vi "Drive Encoder Limit.vi"(0 "MotorControlDevRef":T1, 5 "MotorControlDevRef 2":T1, 7 "MotorControlDevRef 3":T1, 9 "MotorControlDevRef 4":T1, 11 "Limit":dbl, 12 "Invert":bool) -> (4 "MotorControlDevRef out":T1, 6 "MotorControlDevRef out 2":T1, 8 "MotorControlDevRef out 3":T1, 10 "MotorControlDevRef out 4":T1, 15 "Limit Triggered":bool)   [LabVIEW 2019]
uses:
  <vilib>/Rock Robotics/WPI/MotorControl/WPI_MotorControlDeviceRef.ctl
  <vilib>/Rock Robotics/WPI/MotorControl/WPI_MotorControlType.ctl
  <vilib>/Rock Robotics/SystemInterfaces/DIO/FPGA_DIOPWMChannel.ctl
  <vilib>/Rock Robotics/WPI/PWM/WPI_PWMDeadband.ctl
  <vilib>/Rock Robotics/SystemInterfaces/DIO/FPGA_DIOChannel.ctl
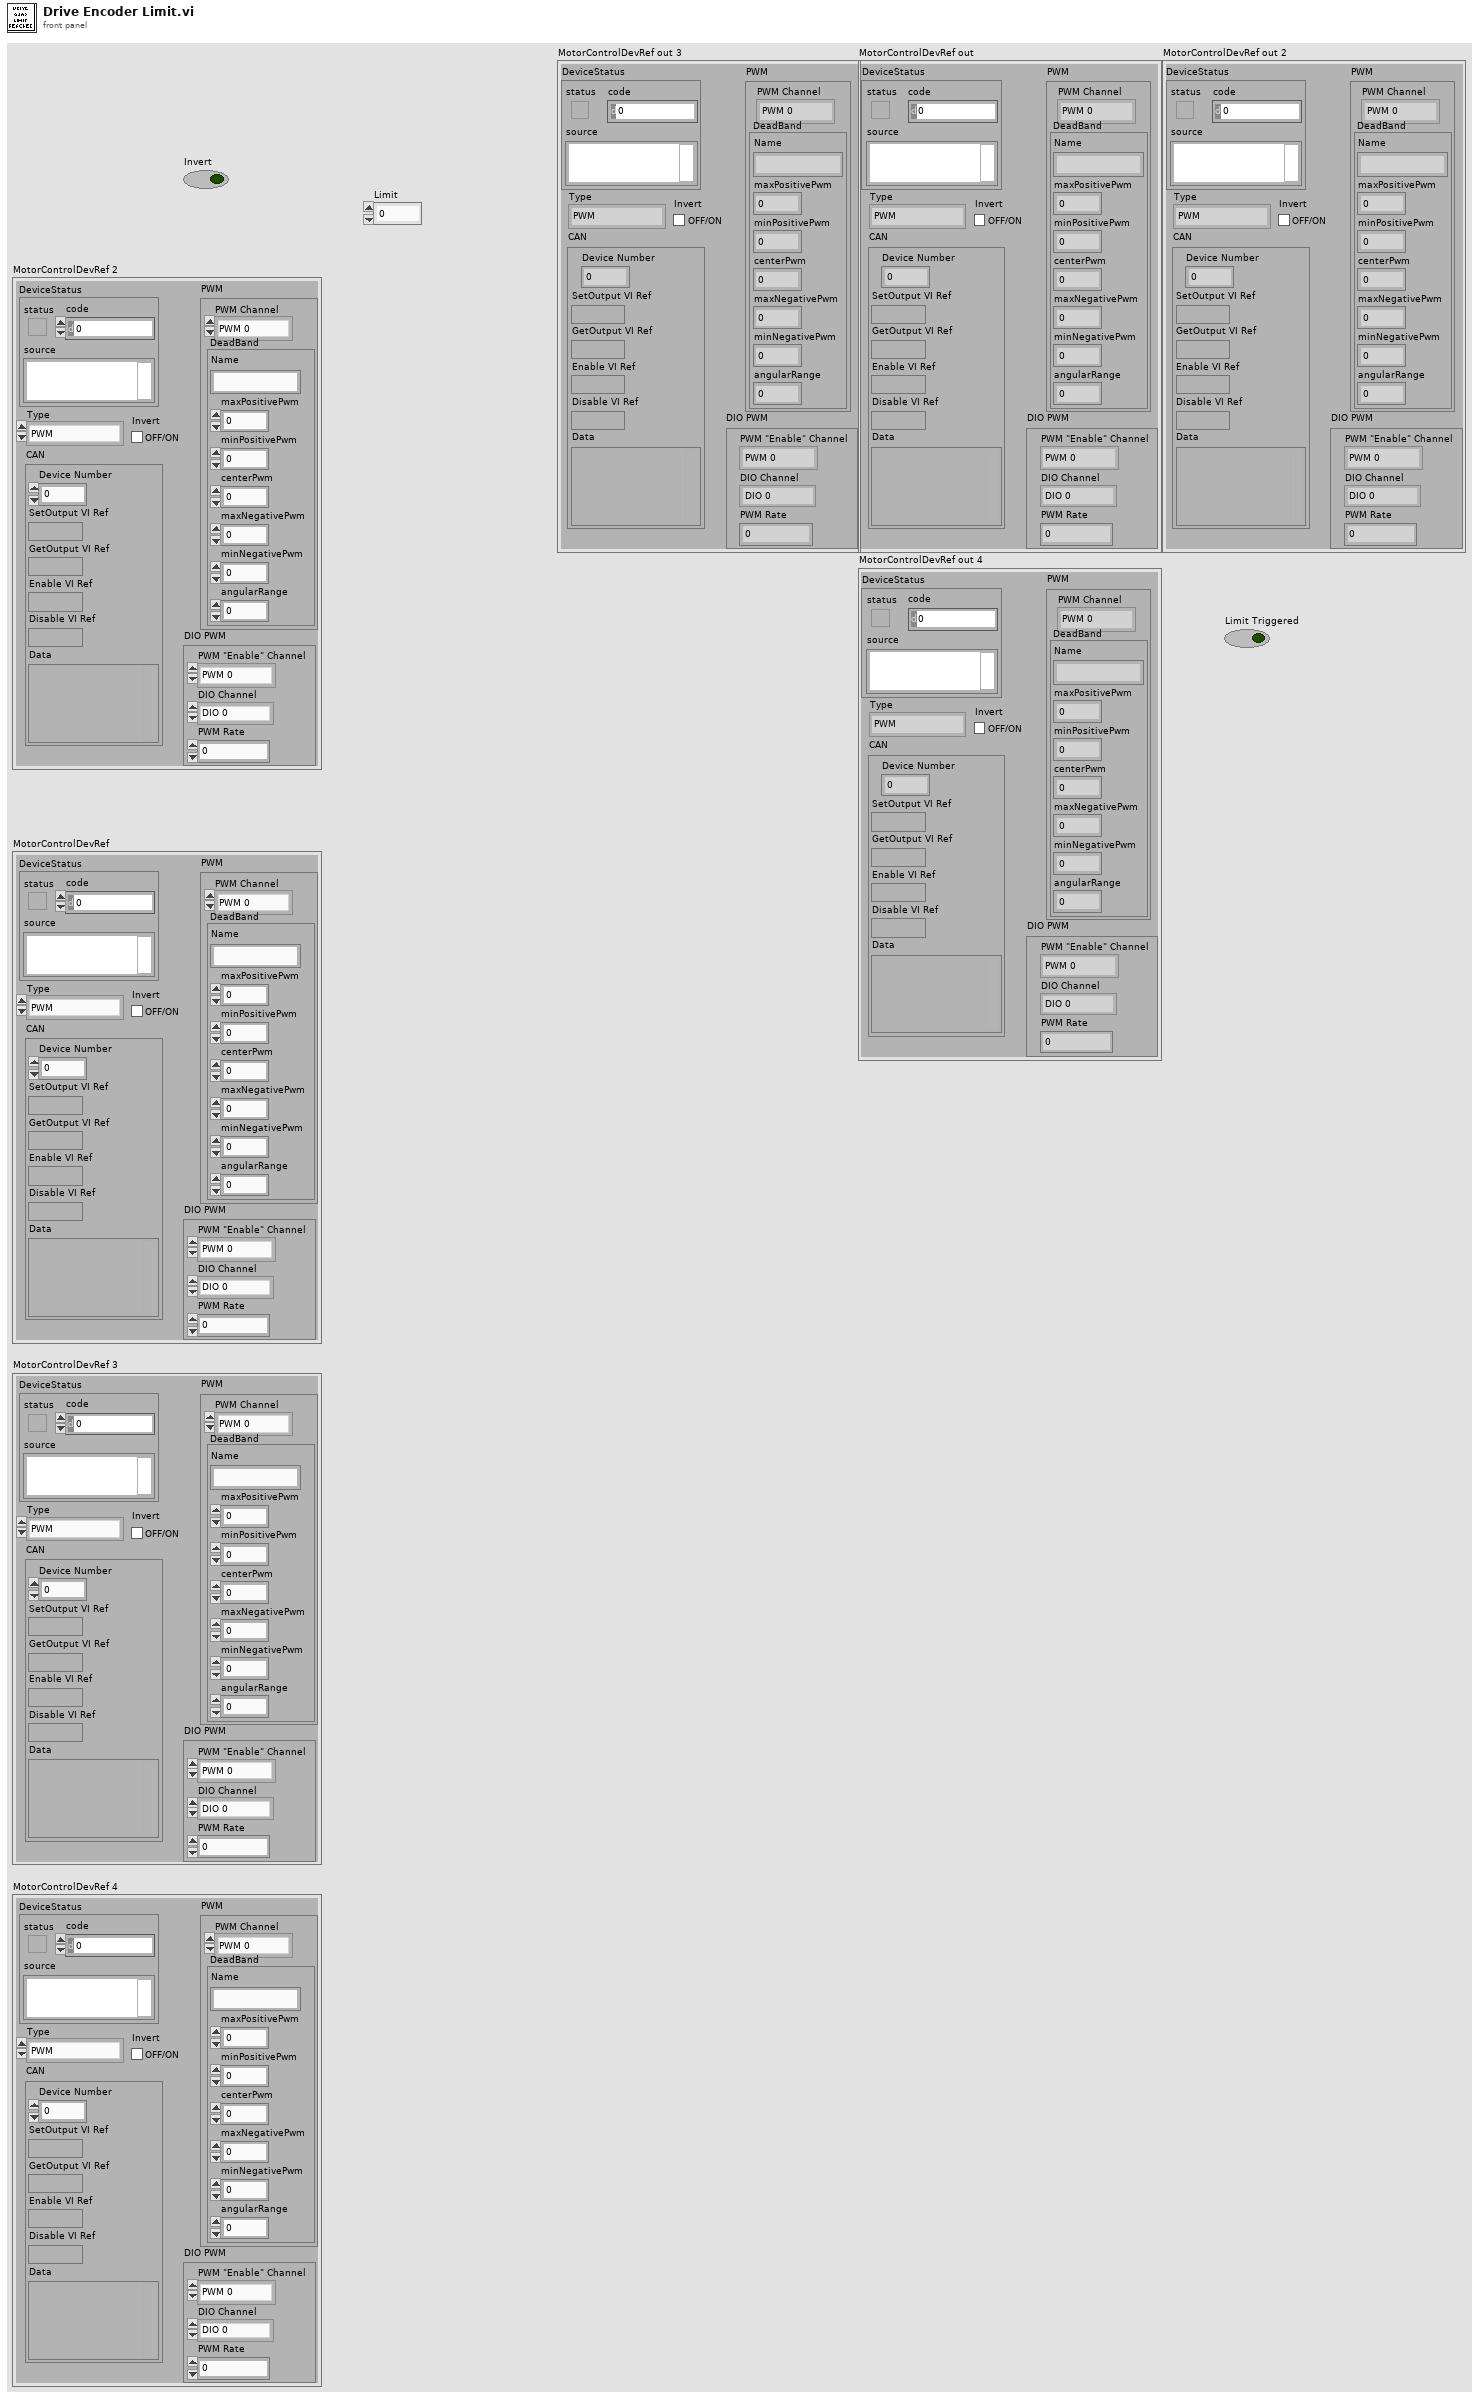
[diagram p1: front panel]
types:
  T1 = typedef "WPI_MotorControlDeviceRef.ctl" = cluster{"DeviceStatus":errorcluster, "Type":T2, "PWM":cluster{"PWM Channel":T3, "DeadBand":T4}, "CAN":cluster{"Device Number":u8, "SetOutput VI Ref":variant, "GetOutput VI Ref":variant, "Enable VI Ref":variant, "Disable VI Ref":variant, "Data":variant}, "Invert":bool, "DIO PWM":cluster{"PWM \"Enable\" Channel":T3, "DIOChannel":T5, "PWM Rate":dbl}}
  T2 = typedef "WPI_MotorControlType.ctl" = enum16{"PWM", "CAN", "DIO PWM"}
  T3 = typedef "FPGA_DIOPWMChannel.ctl" = enum8{"PWM 0", "PWM 1", "PWM 2", "PWM 3", "PWM 4", "PWM 5", "PWM 6", "PWM 7", "PWM 8", "PWM 9", "PWM MXP 0", "PWM MXP 1", "PWM MXP 2", "PWM MXP 3", "PWM MXP 4", "PWM MXP 5", "PWM MXP 6", "PWM MXP 7", "PWM MXP 8", "PWM MXP 9", "Invalid"}
  T4 = typedef "WPI_PWMDeadband.ctl" = cluster{"Name":string, "maxPositivePwm":i32, "minPositivePwm":i32, "centerPwm":i32, "maxNegativePwm":i32, "minNegativePwm":i32, "angularRange":u16}
  T5 = typedef "FPGA_DIOChannel.ctl" = enum8{"DIO 0", "DIO 1", "DIO 2", "DIO 3", "DIO 4", "DIO 5", "DIO 6", "DIO 7", "DIO 8", "DIO 9", "DIO MXP 0", "DIO MXP 1", "DIO MXP 2", "DIO MXP 3", "DIO MXP 4", "DIO MXP 5", "DIO MXP 6", "DIO MXP 7", "DIO MXP 8", "DIO MXP 9", "DIO MXP 10", "DIO MXP 11", "DIO MXP 12", "DIO MXP 13", "DIO MXP 14", "DIO MXP 15", "SPI Port CS1", "SPI Port CS2", "SPI Port CS3", "SPI Port MISO", "SPI Port MOSI", "Invalid"}
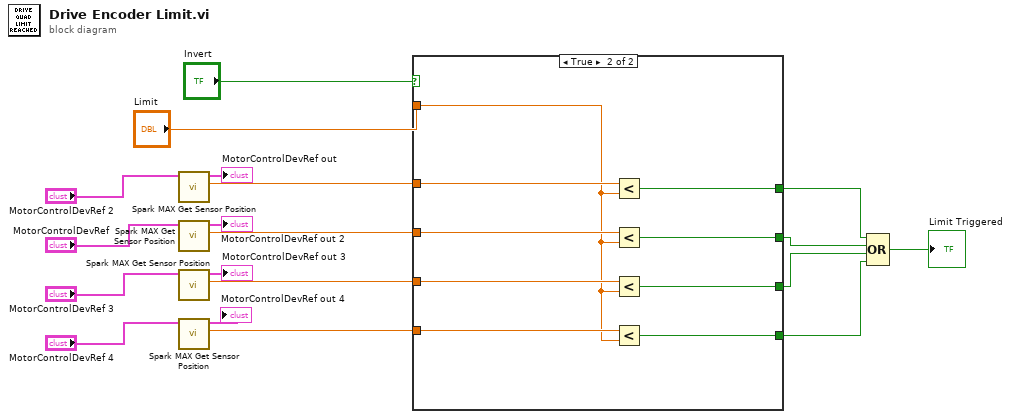
[diagram p0: block diagram]
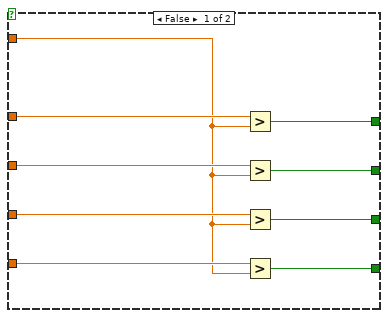
[diagram p2: hidden frame]
diagram:
  n1 = call <vilib>:"Spark MAX Get Sensor Position.vi"("MotorControlDevRef in"="MotorControlDevRef 2") -> ("Sensor Position"=w10:dbl, "MotorControlDevRef out"=→"MotorControlDevRef out":T1)  [unwired: 7 in, 2 out]
  n2 = call <vilib>:"Spark MAX Get Sensor Position.vi"("MotorControlDevRef in"="MotorControlDevRef") -> ("Sensor Position"=w11:dbl, "MotorControlDevRef out"=→"MotorControlDevRef out 2":T1)  [unwired: 7 in, 2 out]
  n3 = call <vilib>:"Spark MAX Get Sensor Position.vi"("MotorControlDevRef in"="MotorControlDevRef 3") -> ("Sensor Position"=w12:dbl, "MotorControlDevRef out"=→"MotorControlDevRef out 3":T1)  [unwired: 7 in, 2 out]
  n4 = call <vilib>:"Spark MAX Get Sensor Position.vi"("MotorControlDevRef in"="MotorControlDevRef 4") -> ("Sensor Position"=w13:dbl, "MotorControlDevRef out"=→"MotorControlDevRef out 4":T1)  [unwired: 7 in, 2 out]
  n5 = case shown="True" "Invert" {
    tunnel: w10 -> [w28 w34]
    tunnel: w11 -> [w27 w35]
    tunnel: w12 -> [w26 w36]
    tunnel: w13 -> [w25 w37]
    tunnel: [w24 w30] -> w14
    tunnel: [w23 w31] -> w15
    tunnel: [w22 w32] -> w16
    tunnel: [w21 w33] -> w17
    tunnel: "Limit" -> [w20 w29]
    frame False {
      n6 = Greater?(x=w28, y=w20) -> (0:w24:bool)
      n7 = Greater?(x=w27, y=w20) -> (0:w23:bool)
      n8 = Greater?(x=w26, y=w20) -> (0:w22:bool)
      n9 = Greater?(x=w25, y=w20) -> (0:w21:bool)
    }
    frame True {
      n10 = Less?(x=w34, y=w29) -> (x < y?=w30:bool)
      n11 = Less?(x=w35, y=w29) -> (x < y?=w31:bool)
      n12 = Less?(x=w36, y=w29) -> (x < y?=w32:bool)
      n13 = Less?(x=w37, y=w29) -> (x < y?=w33:bool)
    }
  }
  n14 = Compound Arithmetic op=OR(w14, w15, w16, w17) -> (→"Limit Triggered":bool)
